vi "Get Window Size.vi"(11 "Window Bounds":T2) -> (3 "Window Size":T1)   [LabVIEW 2019, in "Window.lvlib"]
doc: "Gets the horizontal and vertical dimensions of a given bounding rectangle. Result will be in pixels."
uses:
  Window.lvlib
  _2D/Point.ctl
  _2D/2D.lvlib
  <vilib>/Utility/miscctls.llb/LVRectTypeDef.ctl
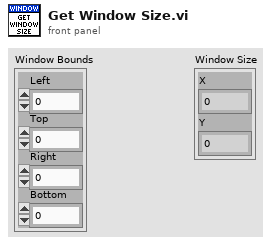
[diagram p1: front panel]
types:
  T1 = typedef "2D.lvlib/Point.ctl" = cluster{"X":i16, "Y":i16}
  T2 = typedef "LVRectTypeDef.ctl" = cluster{"Left":i16, "Top":i16, "Right":i16, "Bottom":i16}
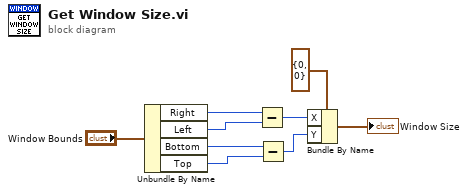
[diagram p0: block diagram]
diagram:
  n1 = Unbundle By Name("Window Bounds") -> ("Right"=w8:i16, "Left"=w7:i16, "Bottom"=w4:i16, "Top"=w3:i16)
  n2 = Subtract(x=w8, y=w7) -> (x-y=w5:i16)
  n3 = Subtract(x=w4, y=w3) -> (x-y=w2:i16)
  n4 = Bundle By Name(cluster=T1 {"X"=0, "Y"=0} ("Window Size"), "X"=w5, "Y"=w2) -> (→"Window Size":T1)
